vi "Generate RPC Messages.vi"(7 "Messages MetaData":T1[](array[typedef]), 8 "error in (no error)":errorcluster, 11 "LVClassLibrary in":refnum<vi>) -> (0 "error out":errorcluster, 3 "LVClassLibrary out":refnum<vi>)   [LabVIEW 2019, in "gRPC Scripting Tools.lvlib"]
uses:
  gRPC Scripting Tools.lvlib
  TypeDefs/Message Metadata (Scripting).ctl
  TypeDefs/Message Element Metadata (Scripting).ctl
  TypeDefs/Message Element Type.ctl
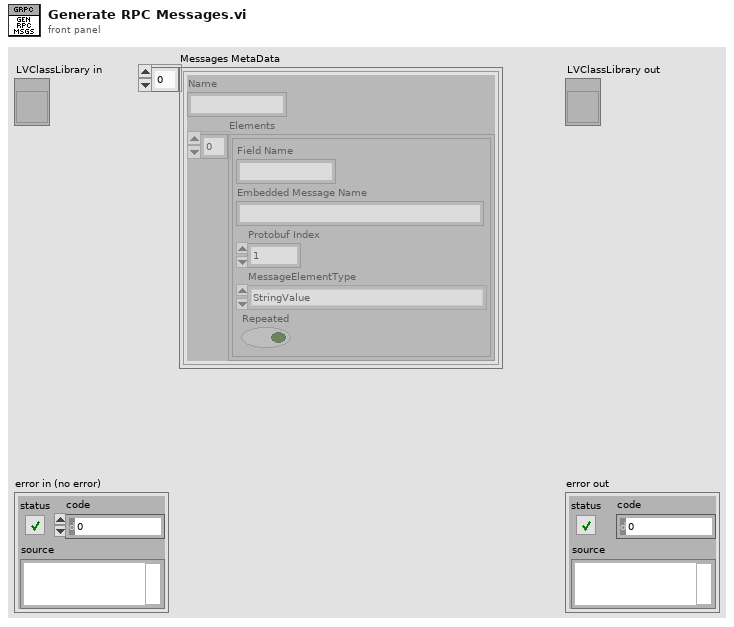
[diagram p1: front panel]
types:
  T1 = typedef "gRPC Scripting Tools.lvlib/Message Metadata (Scripting).ctl" = cluster{"Name":string, "Elements":T2[]}
  T2 = typedef "gRPC Scripting Tools.lvlib/Message Element Metadata (Scripting).ctl" = cluster{"Field Name":string, "Embedded Message Name":string, "Protobuf Index":i32, "MessageElementType":T3, "Repeated":bool}
  T3 = typedef "gRPC Scripting Tools.lvlib/Message Element Type.ctl" = enum32{"Int32Value", "FloatValue", "DoubleValue", "BoolValue", "StringValue", "MessageValue", ""}
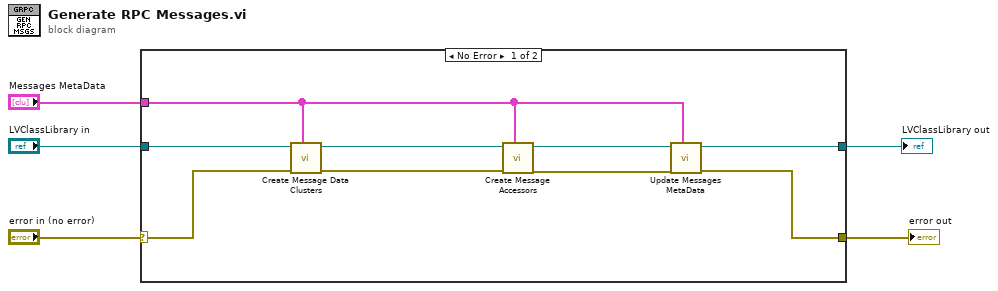
[diagram p0: block diagram]
diagram:
  n1 = case shown="No Error" "error in (no error)" {
    selector: "error in (no error)" -> [w7 w15]
    tunnel: [w14 w15] -> w5
    tunnel: [w13 w16] -> w4
    tunnel: "LVClassLibrary in" -> [w12 w16]
    tunnel: "Messages MetaData" -> [w6 _]
    frame No Error {
      n2 = call "Create Message Data Clusters.vi"("Message parameters"=w6, "error in (no error)"=w7, "Server class in"=w12) -> ("error out"=w8:errorcluster, "Server class out"=w9:refnum<vi>)  [unwired: 7 in]
      n3 = call "Create Message Accessors.vi"("Message parameters"=w6, "error in (no error)"=w8, "Server class in"=w9) -> ("error out"=w11:errorcluster, "Server class out"=w10:refnum<vi>)  [unwired: 7 in]
      n4 = call "Update Messages MetaData.vi"("Messages MetaData"=w6, "error in (no error)"=w11, "LVClassLibrary in"=w10) -> ("error out"=w14:errorcluster, "LVClassLibrary out"=w13:refnum<vi>)  [unwired: 7 in]
    }
    frame Error {
    }
  }
  "error out" <- w5
  "LVClassLibrary out" <- w4
